vi "CircularCycle.vi"(9 "Reset Cycle":bool caption="Reset Cycle (F)", 10 "n":i32 min=0) -> (2 "Circular Cycle":i32)   [LabVIEW 2017, in "GPNumeric.lvlib"]
doc: "Outputs a cyclic number on <B>Circular Cycle</B> when called repeatedly.\n\nThe cycle for this VI is 0, 1, 2 ... <B>n</B>, and then it starts over.\n\nThis can be useful when implementing a circular buffer for instance.\n\nSetting <B>Reset Cycle</B> to True makes <B>Circular Cycle</B> start from 0 again.\n\nThis VI is inlined.\n\nSteen Schmidt\nGPower\n7/4 2014"
uses:
  GPNumeric.lvlib
panel:
  # "Copyright © 2014\nGPower\nSee enclosed license file for terms and conditions"
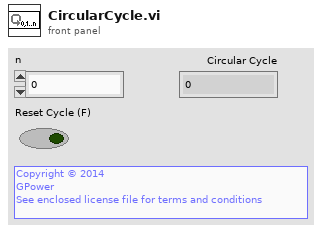
[diagram p1: front panel]
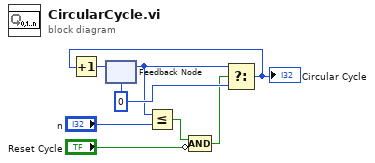
[diagram p0: block diagram]
diagram:
  w6 = 0
  n1 = feedback #1(w6) -> (w5:i32)
  n2 = Less Or Equal?(x=w5, y="n") -> (x <= y?=w2:bool)
  n3 = Compound Arithmetic op=AND(w2, invert "Reset Cycle") -> (w1:bool)
  n4 = Select(t=w5, s=w1, f=w6) -> (s? t:f=w8:i32)
  "Circular Cycle" <- w8
  n5 = Increment(x=w8) -> (x+1=w7:i32)
  n6 = feedback-in #1(w7) -> ()
